vi "Untitled 3.vi"() -> ()   [LabVIEW 2014]
panel:
  out "switch_control_json":string
  out "switch_data_json":string
  out "train_control_json":string
  out "train_data_json":string
  out "train_data_out":T1
  out "switch_control_out":T2
  out "switch_data_out":T3
  out "train_control_out":T4
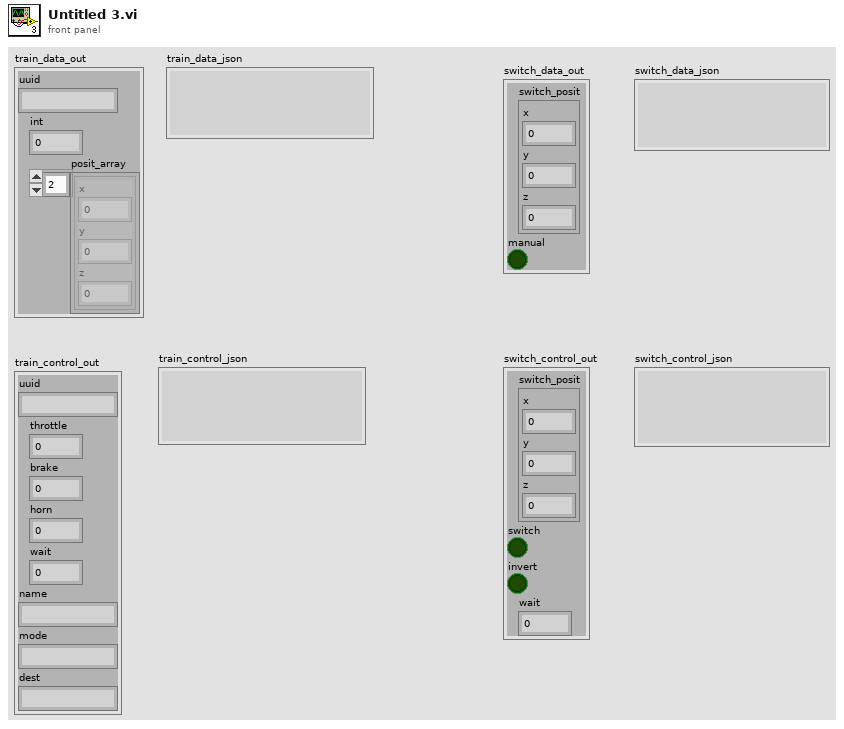
[diagram p1: front panel]
types:
  T1 = cluster{"uuid":string, "int":i32, "posit_array":cluster{"x":dbl, "y":dbl, "z":dbl}[]}
  T2 = cluster{"switch_posit":cluster{"x":dbl, "y":dbl, "z":dbl}, "switch":bool, "invert":bool, "wait":dbl}
  T3 = cluster{"switch_posit":cluster{"x":dbl, "y":dbl, "z":dbl}, "manual":bool}
  T4 = cluster{"uuid":string, "throttle":dbl, "brake":dbl, "horn":dbl, "wait":dbl, "name":string, "mode":string, "dest":string}
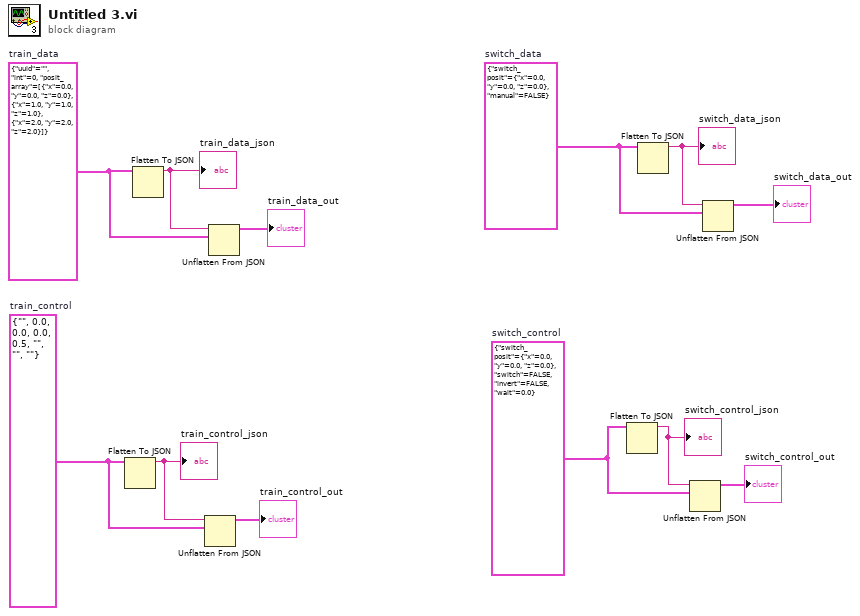
[diagram p0: block diagram]
diagram:
  w5 = T2 {"switch_posit"={"x"=0.0, "y"=0.0, "z"=0.0}, "switch"=FALSE, "invert"=FALSE, "wait"=0.0}  # switch_control
  w4 = T3 {"switch_posit"={"x"=0.0, "y"=0.0, "z"=0.0}, "manual"=FALSE}  # switch_data
  w9 = T4 {"uuid"="", "throttle"=0.0, "brake"=0.0, "horn"=0.0, "wait"=0.5, "name"="", "mode"="", "dest"=""}  # train_control
  w12 = T1 {"uuid"="", "int"=0, "posit_array"=[{"x"=0.0, "y"=0.0, "z"=0.0}, {"x"=1.0, "y"=1.0, "z"=1.0}, {"x"=2.0, "y"=2.0, "z"=2.0}]}  # train_data
  n1 = Flatten To JSON(anything=w9) -> (JSON string=w10:string)  [unwired: 2 in, 1 out]
  "train_control_json" <- w10
  n2 = Flatten To JSON(anything=w12) -> (JSON string=w11:string)  [unwired: 2 in, 1 out]
  "train_data_json" <- w11
  n3 = Unflatten From JSON(JSON string=w10, type and defaults=w9) -> (value=→"train_control_out":T4)  [unwired: 5 in, 1 out]
  n4 = Unflatten From JSON(JSON string=w11, type and defaults=w12) -> (value=→"train_data_out":T1)  [unwired: 5 in, 1 out]
  n5 = Flatten To JSON(anything=w5) -> (JSON string=w6:string)  [unwired: 2 in, 1 out]
  "switch_control_json" <- w6
  n6 = Flatten To JSON(anything=w4) -> (JSON string=w7:string)  [unwired: 2 in, 1 out]
  "switch_data_json" <- w7
  n7 = Unflatten From JSON(JSON string=w6, type and defaults=w5) -> (value=→"switch_control_out":T2)  [unwired: 5 in, 1 out]
  n8 = Unflatten From JSON(JSON string=w7, type and defaults=w4) -> (value=→"switch_data_out":T3)  [unwired: 5 in, 1 out]
